vi "Anritsu VNA Unflatten Driver Configuration.vi"(9 "VNA Configuration (\"\")":string) -> (1 "Configuration":T1={"BusType"=enum."GPIB", "GPIB Bus"=0, "GPIB Address"=0, "IP"=0, "COM"=0, "Baud Rate"=enum."300", "USB Device"=0, "Instrument S\\N"="", "SCIL Address"=16} {"USB Device" max=31 step=1}, 4 "Version":string)   [LabVIEW 2011]
uses:
  VNA Configuration.ctl
  VNA Configuration v2.ctl
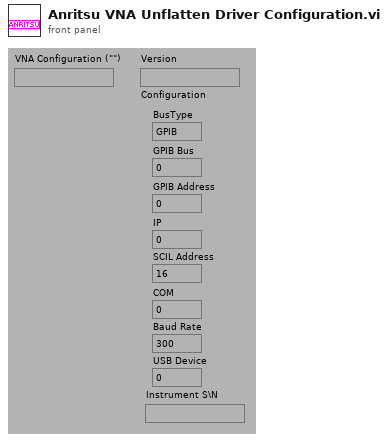
[diagram p1: front panel]
types:
  T1 = typedef "VNA Configuration.ctl" = cluster{"BusType":enum32{"GPIB", "LAN/IP", "Serial", "USB"}, "GPIB Bus":i32, "GPIB Address":i32, "IP":u32, "COM":i32, "Baud Rate":enum32{"300", "600", "1200", "2400", "4800", "9600"}, "USB Device":u32, "Instrument S\\N":string, "SCIL Address":i32}
  T2 = typedef "VNA Configuration v2.ctl" = cluster{"BusType":enum32{"GPIB", "LAN/IP", "Serial", "USB"}, "GPIB Bus":i32, "GPIB Address":i32, "IP":u32, "COM":i32, "Baud Rate":enum32{"300", "600", "1200", "2400", "4800", "9600"}, "USB Device":u32, "Instrument S\\N":string}
  T3 = enum32{"300", "600", "1200", "2400", "4800", "9600"}
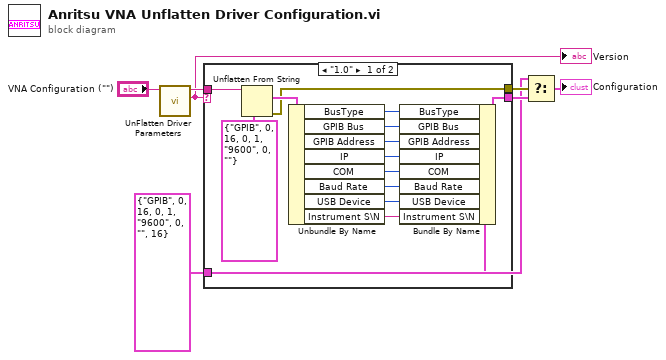
[diagram p0: block diagram]
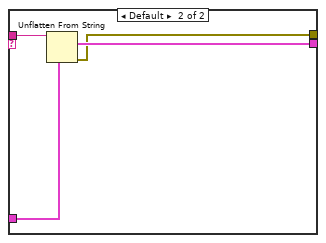
[diagram p2: hidden frame]
diagram:
  w2 = T1 {"BusType"=enum."GPIB", "GPIB Bus"=0, "GPIB Address"=16, "IP"=0, "COM"=1, "Baud Rate"=enum."9600", "USB Device"=0, "Instrument S\\N"="", "SCIL Address"=16} ("Configuration")
  n1 = call "UnFlatten Driver Parameters.vi"("Flattened Driver Parameters with Version (\"\")"="VNA Configuration (\"\")") -> ("Driver Version"=w1:string, "Flat Driver Parameters"=w3:string)  [unwired: 1 in, 4 out]
  "Version" <- w1
  n2 = case shown="\"1.0\"" w1 {
    tunnel: [w18 w25] -> w7
    tunnel: [w8 w22] -> w5
    tunnel: w3 -> [w21 w24]
    tunnel: w2 -> [w19 w23]
    frame "1.0" {
      n3 = Unflatten From String(type=T2 {"BusType"=enum."GPIB", "GPIB Bus"=0, "GPIB Address"=16, "IP"=0, "COM"=1, "Baud Rate"=enum."9600", "USB Device"=0, "Instrument S\\N"=""} ("Configuration"), binary string=w21) -> (value=w17:T2, error out=w8:errorcluster)  [unwired: 1 in, 3 out]
      n4 = Unbundle By Name(w17) -> ("BusType"=w16:enum32{"GPIB", "LAN/IP", "Serial", "USB"}, "GPIB Bus"=w15:i32, "GPIB Address"=w14:i32, "IP"=w13:u32, "COM"=w12:i32, "Baud Rate"=w11:T3, "USB Device"=w10:u32, "Instrument S\\N"=w9:string)
      n5 = Bundle By Name(cluster=w19, "BusType"=w16, "GPIB Bus"=w15, "GPIB Address"=w14, "IP"=w13, "COM"=w12, "Baud Rate"=w11, "USB Device"=w10, "Instrument S\\N"=w9) -> (w18:T1)
    }
    frame Default {
      n6 = Unflatten From String(type=w23, binary string=w24) -> (value=w25:T1, error out=w22:errorcluster)  [unwired: 1 in, 3 out]
    }
  }
  n7 = Select(t=w2, s=w5, f=w7) -> (s? t:f=→"Configuration":T1)
